vi "Parse Available Assets.vi"(8 "error in (no error)":errorcluster, 9 "server url in":string, 10 "Statistics in":T2, 11 "Refnum in":T1) -> (0 "error out":errorcluster, 2 "Statistics out":T2, 3 "Refnum out":T1)   [LabVIEW 2020]
uses:
  <vilib>/httpClient/ClientHandle.ctl
  <vilib>/httpClient/LabVIEWHTTPClient.lvlib
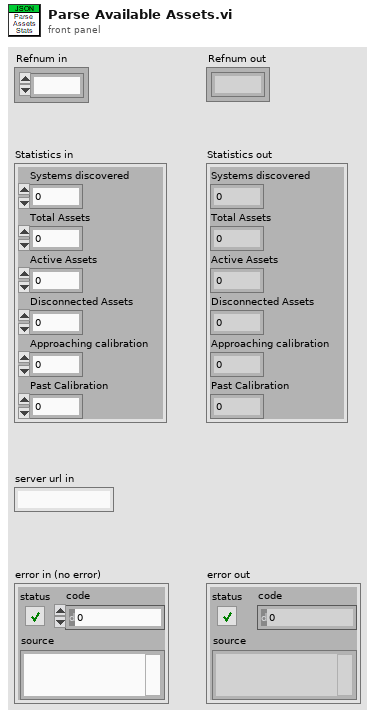
[diagram p1: front panel]
types:
  T1 = typedef "LabVIEWHTTPClient.lvlib/ClientHandle.ctl" = refnum<k1>
  T2 = cluster{"Systems discovered":i32, "Total Assets":i32, "Active Assets":i32, "Disconnected Assets":i32, "Approaching calibration ":i32, "Past Calibration":i32}
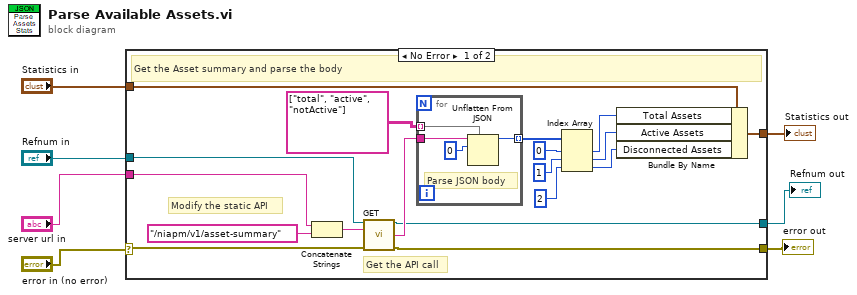
[diagram p0: block diagram]
diagram:
  n1 = case shown="No Error" "error in (no error)" {
    selector: "error in (no error)" -> [w8 w32]
    tunnel: [w25 w31] -> w7
    tunnel: "Statistics in" -> [w17 w31]
    tunnel: "server url in" -> [w14 _]
    tunnel: "Refnum in" -> [w11 w30]
    tunnel: [w10 w30] -> w2
    tunnel: [w9 w32] -> w1
    frame No Error {
      # "Get the API call"
      # "Modify the static API"
      # "Get the Asset summary and parse the body"
      n2 = Concatenate Strings(w14, "/niapm/v1/asset-summary" ("Get Asset count API")) -> (w13:string)
      n3 = call <vilib>:"GET.vi"("client handle"=w11, "url"=w13, "error in (no error)"=w8) -> ("client handle out"=w10:T1, "body"=w15:string, "error out"=w9:errorcluster)  [unwired: 9 in, 1 out]
      n4 = for {
        tunnel: w15 -> [w29]
        tunnel: string[][] [["total"], ["active"], ["notActive"]] -> [w27] mode=indexing
        tunnel: [w26] -> w18 mode=indexing
        # "Parse JSON body"
        n5 = Unflatten From JSON(path=w27, JSON string=w29, type and defaults=0) -> (value=w26:i32)  [unwired: 4 in, 1 out]
      }
      n6 = Index Array(array=w18, index #1=0 ("index"), index #2=1 ("index"), index #3=2 ("index")) -> (element #1=w22:i32, element #2=w23:i32, element #3=w24:i32)
      n7 = Bundle By Name(cluster=w17, "Total Assets"=w22, "Active Assets"=w23, "Disconnected Assets"=w24) -> (w25:T2)
    }
    frame Error {
    }
  }
  "Statistics out" <- w7
  "Refnum out" <- w2
  "error out" <- w1
